vi "initiate.vi"(8 "error in (no error)":errorcluster, 11 "reference in":refnum<class "Master Controller.lvclass">) -> (0 "error out":errorcluster, 3 "reference out":refnum<class "Master Controller.lvclass">)   [LabVIEW 2015, in "Master Controller.lvclass"]
uses:
  Master Controller.lvclass
  File Controller_llb/File Controller.lvclass
  Devices Controller_llb/Devices Controller.lvclass
  Items Controller_llb/Items Controller.lvclass
  GUI/GUI Controller_llb/GUI Controller.lvclass
  Notification Controller_class/Notification Controller.lvclass
  PartsTracking Controller_class/PartsTracking Controller.lvclass
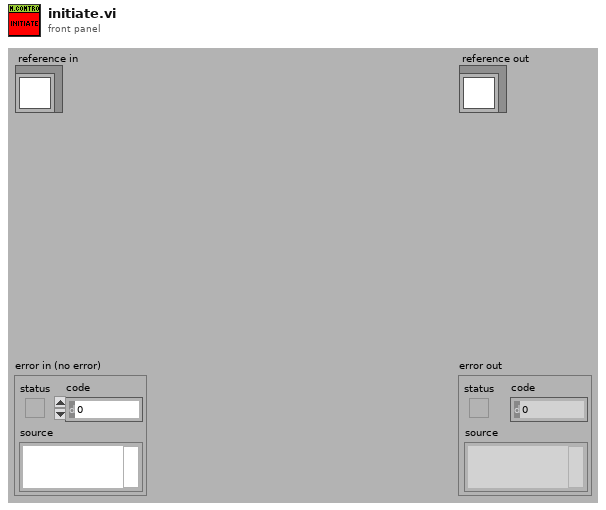
[diagram p1: front panel]
types:
  T1 = typedef "Master Controller.lvclass/ObjectAttributesRef.ctl" = refnum<data-value>
  T2 = typedef "Master Controller.lvclass/ObjectAttributes.ctl" = cluster{"MyAttribute":dbl, "Devices Controller_ref":refnum<class "Devices Controller.lvclass">, "File Controller_ref":refnum<class "File Controller.lvclass">, "Items Controller_ref":refnum<class "Items Controller.lvclass">, "GUI Controller_ref":refnum<class "GUI Controller.lvclass">, "NotificationController_ref":refnum<class "Notification Controller.lvclass">, "PartsTracking Controller_ref":refnum<class "PartsTracking Controller.lvclass">}
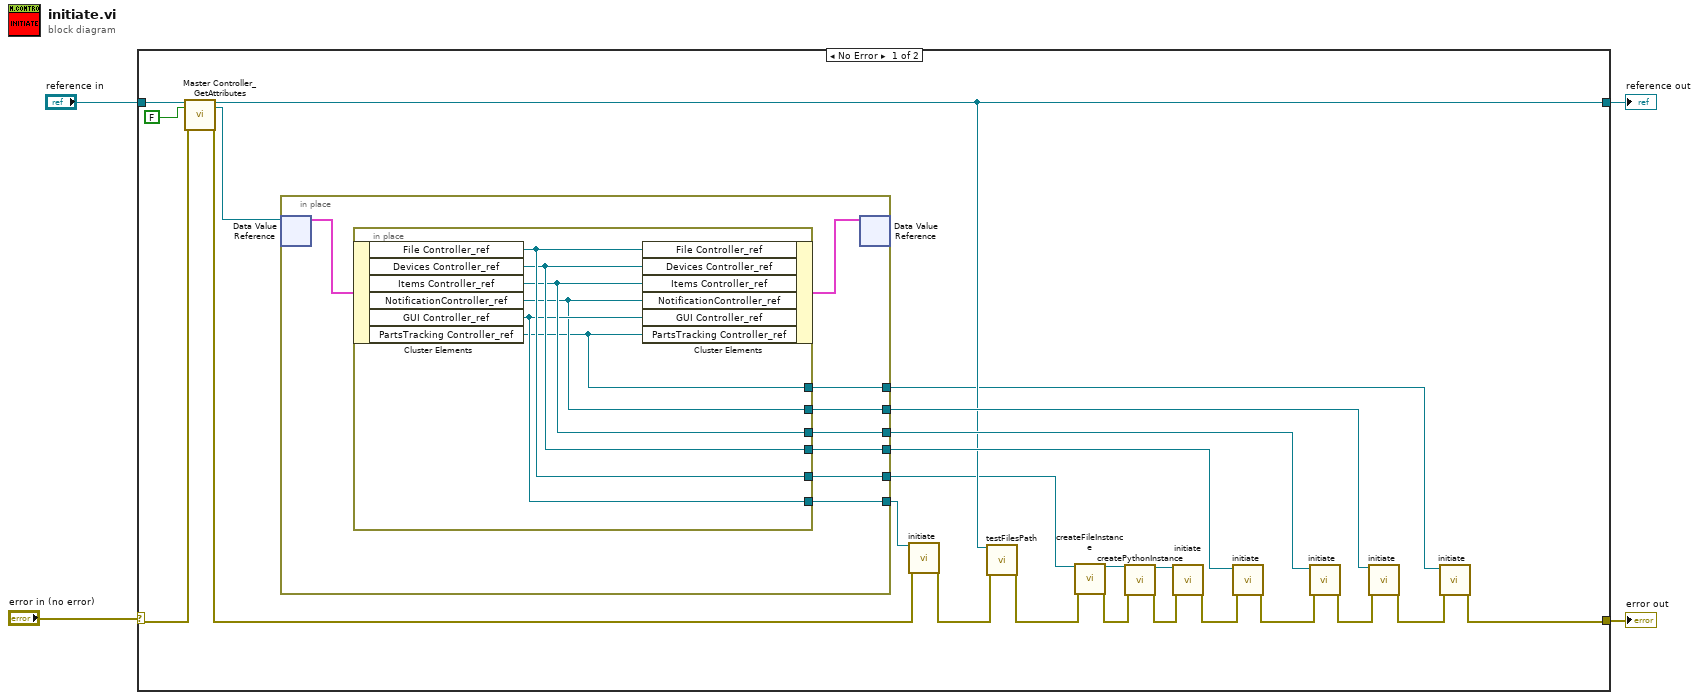
[diagram p0: block diagram]
diagram:
  n1 = case shown="No Error" "error in (no error)" {
    selector: "error in (no error)" -> [w25 w43]
    tunnel: [w10 w43] -> w3
    tunnel: [w16 w42] -> w1
    tunnel: "reference in" -> [w27 w42]
    frame No Error {
      n2 = call "Master Controller_GetAttributes.vi"("reference in"=w27, "return data? (T)"=FALSE, "error in (no error)"=w25) -> ("reference out"=w16:refnum<class "Master Controller.lvclass">, "attributes ref"=w24:T1, "error out"=w17:errorcluster)  [unwired: 13 in, 1 out]
      n3 = in-place {
        in-place-border: [w33] -> w14
        in-place-border: [w32] -> w23
        in-place-border: [w31] -> w20
        in-place-border: [w30] -> w19
        in-place-border: [w29] -> w18
        in-place-border: [w28] -> w12
        n4 = in-place-dvr #1(w24) -> (w34:T2)  [unwired: 1 out]
        n5 = in-place {
          in-place-border: [w41] -> w33
          in-place-border: [w40] -> w32
          in-place-border: [w39] -> w31
          in-place-border: [w38] -> w30
          in-place-border: [w37] -> w29
          in-place-border: [w36] -> w28
          n6 = in-place-cluster #2(w34) -> ("File Controller_ref"=w41:refnum<class "File Controller.lvclass">, "Devices Controller_ref"=w40:refnum<class "Devices Controller.lvclass">, "Items Controller_ref"=w39:refnum<class "Items Controller.lvclass">, "NotificationController_ref"=w37:refnum<class "Notification Controller.lvclass">, "GUI Controller_ref"=w38:refnum<class "GUI Controller.lvclass">, "PartsTracking Controller_ref"=w36:refnum<class "PartsTracking Controller.lvclass">)
          n7 = in-place-cluster #2("File Controller_ref"=w41, "Devices Controller_ref"=w40, "Items Controller_ref"=w39, "NotificationController_ref"=w37, "GUI Controller_ref"=w38, "PartsTracking Controller_ref"=w36) -> (w35:T2)
        }
        n8 = in-place-dvr #1(w35) -> ()  [unwired: 2 out]
      }
      n9 = call "initiate.vi"("reference in"=w19, "error in (no error)"=w17) -> ("error out"=w15:errorcluster)  [unwired: 16 in, 1 out]
      n10 = call "testFilesPath.vi"("reference in"=w16, "error in (no error)"=w15) -> ("error out"=w13:errorcluster)  [unwired: 16 in, 1 out]
      n11 = call "createFileInstance.vi"("reference in"=w14, "error in (no error)"=w13) -> ("reference out"=w8:refnum<class "File Controller.lvclass">, "error out"=w7:errorcluster)  [unwired: 16 in]
      n12 = call "createPythonInstance.vi"("reference in"=w8, "error in (no error)"=w7) -> ("reference out"=w5:refnum<class "File Controller.lvclass">, "error out"=w6:errorcluster)  [unwired: 16 in]
      n13 = call "initiate.vi"("reference in"=w5, "error in (no error)"=w6) -> ("error out"=w22:errorcluster)  [unwired: 16 in, 1 out]
      n14 = call "initiate.vi"("error in (no error)"=w22, "reference in"=w23) -> ("error out"=w21:errorcluster)  [unwired: 8 in, 1 out]
      n15 = call "initiate.vi"("error in (no error)"=w21, "reference in"=w20) -> ("error out"=w9:errorcluster)  [unwired: 8 in, 1 out]
      n16 = call "initiate.vi"("reference in"=w18, "error in (no error)"=w9) -> ("error out"=w11:errorcluster)  [unwired: 16 in, 1 out]
      n17 = call "initiate.vi"("error in (no error)"=w11, "reference in"=w12) -> ("error out"=w10:errorcluster)  [unwired: 8 in, 1 out]
    }
    frame Error {
    }
  }
  "error out" <- w3
  "reference out" <- w1
